vi "LVClass_HasoField Get Wavelenght.vi"(0 "HasoField in":refnum<class "HasoField.lvclass">, 11 "error in (no error)":errorcluster) -> (4 "HasoField out":refnum<class "HasoField.lvclass">, 8 "wavelenght":dbl, 15 "error out":errorcluster)   [LabVIEW 2020, in "HasoField.lvclass"]
doc: "Get the wavelength of the source.\n\n--------------------------------------------------------------------------------\n\n<B>HasoFieldIn </B> : HasoField object.\n<B>HasoFieldOut </B> : HasoField object.\n<B>wavelength </B> : Wavelength of the source.\n<B>ErrorIn </B> : Error\n<B>ErrorOut </B> : Error\n\n--------------------------------------------------------------------------------"
uses:
  HasoField.lvclass
  HasoField.lvclass/HasoField.ctl
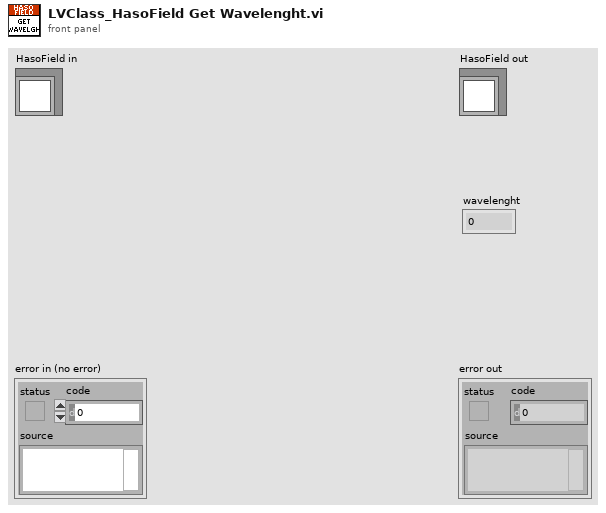
[diagram p1: front panel]
types:
  T1 = typedef "ClassID.ctl" = i64
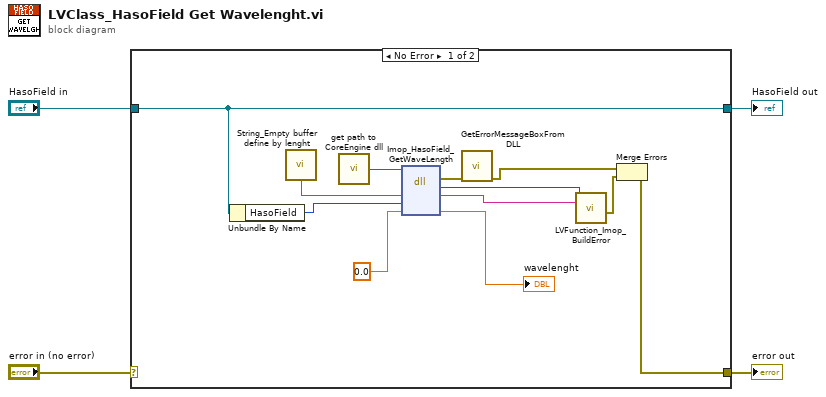
[diagram p0: block diagram]
diagram:
  n1 = case shown="No Error" "error in (no error)" {
    selector: "error in (no error)" -> [_ w18]
    tunnel: [w5 w18] -> w3
    tunnel: [w7 w17] -> w1
    tunnel: "HasoField in" -> [w7 w17]
    frame No Error {
      n2 = Unbundle By Name(w7) -> ("HasoField"=w6:T1)
      n3 = call "String_Empty buffer define by lenght.vi"() -> ("Empty buffer"=w12:string)  [unwired: 1 in]
      n4 = call "get path to CoreEngine dll.vi"() -> ("path to wavekit library"=w11:path)  [unwired: 14 in, 1 out]
      n5 = dll-call lib="D:/soft/HASO_v3/SVN_trunk/ImOpCoreEngine4_LV2011/DLLs/c_interface_vc100.dll" fn="Imop_HasoField_GetWaveLength"(path in=w11, "message"=w12, "HasoField"=w6, "wavelenght"=0.0 ("wavelength")) -> (error out=w10:errorcluster, "return type"=w15:i32, "message"=w16:string, "wavelenght"=→"wavelenght":dbl)  [unwired: 3 in, 1 out]
      n6 = call "GetErrorMessageBoxFromDLL.vi"("error IN"=w10) -> ("error OUT"=w14:errorcluster)  [unwired: 10 in]
      n7 = call "LVFunction_Imop_BuildError.vi"("code"=w15, "String to Prepend to source (\"\")"=w16) -> ("error out"=w13:errorcluster)  [unwired: 13 in]
      n8 = Merge Errors(w14, w13) -> (w5:errorcluster)
    }
    frame Error {
    }
  }
  "error out" <- w3
  "HasoField out" <- w1
